vi "Append Image.vi"(8 "error in (no error)":errorcluster, 10 "Image File Path":path, 11 "Document in":refnum<class "Document.lvclass">) -> (0 "error out":errorcluster, 3 "Document out":refnum<class "Document.lvclass">)   [LabVIEW 2017, in "LabVIEW NPOI.lvlib" / "Document.lvclass"]
doc: "Appends the image located at <b>Image File Path</b> to the <b>Document</b>. Only PNG and JPG format are supported."
uses:
  Document.lvclass
  <vilib>/Utility/error.llb/Error Cluster From Error Code.vi
  <vilib>/ErrorRing/Error Ring.xnode
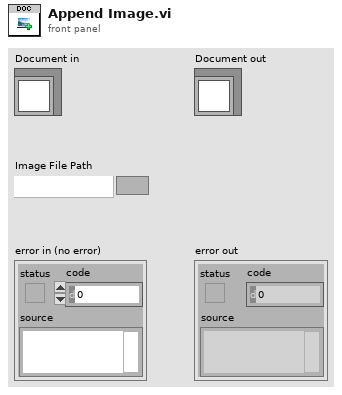
[diagram p1: front panel]
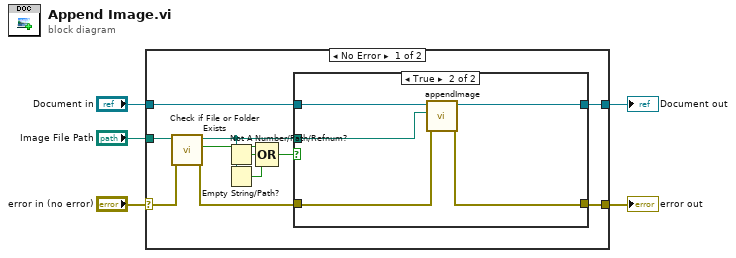
[diagram p0: block diagram]
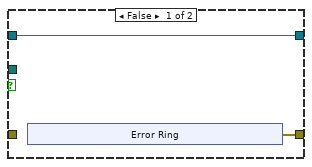
[diagram p2: hidden frame]
diagram:
  n1 = case shown="No Error" "error in (no error)" {
    selector: "error in (no error)" -> [w8 w29]
    tunnel: [w14 w29] -> w4
    tunnel: [w15 w28] -> w2
    tunnel: "Document in" -> [w16 w28]
    tunnel: "Image File Path" -> [w10 _]
    frame No Error {
      n2 = call <vilib>:"Check if File or Folder Exists.vi"("error in (no error)"=w8, "path"=w10) -> ("error out"=w7:errorcluster, "file or folder exists?"=w11:bool, "dup path"=w9:path)  [unwired: 7 in]
      n3 = Not A Number/Path/Refnum?(number/path/refnum=w9) -> (NaN/Path/Refnum?=w13:bool)
      n4 = Empty String/Path?(string/path=w9) -> (empty?=w12:bool)
      n5 = Compound Arithmetic op=OR(w11, w13, w12) -> (w6:bool)
      n6 = case shown="True" w6 {
        tunnel: w16 -> [w18 w27]
        tunnel: [w18 w26] -> w15
        tunnel: [w17 w25] -> w14
        tunnel: w9 -> [_ w24]
        tunnel: w7 -> [_ w23]
        frame False {
          n7 = xnode "Error Ring"() -> ("error out"=w17:errorcluster)
        }
        frame True {
          n8 = call-dynamic "appendImage.vi"("error in (no error)"=w23, "Image Path"=w24, "Document in"=w27) -> ("error out"=w25:errorcluster, "Document out"=w26:refnum<class "Document.lvclass">)  [unwired: 7 in]
        }
      }
    }
    frame Error {
    }
  }
  "error out" <- w4
  "Document out" <- w2
